vi "Initialize Sessions - NSess.vi"(6 "initialize and close session behavior":T1, 7 "option string":string, 8 "error in":errorcluster, 9 "reset":bool, 11 "session reservation in":refnum<class "Session Reservation.lvclass">) -> (0 "error out":errorcluster, 1 "channel lists":string[](array[string]), 2 "sessions":refnum<k15>[](array[refnum]), 3 "session reservation out":refnum<class "Session Reservation.lvclass">)   [LabVIEW 2020, in "MeasurementLink niDigital.lvlib"]
doc: "Create the NI-Digital driver sessions from the <b>session reservation in</b>."
uses:
  MeasurementLink niDigital.lvlib
  b3cb301c-7684-4518-818f-a956a366db36.vi
  Session Factory/Session Factory.lvclass
  Measurements/Measurement Plugin Session Management V1/Session Reservation/Session Reservation.lvclass
  Measurements/Measurement Plugin Session Management V1/Session Reservation/Initialize and Close Session Behavior.ctl
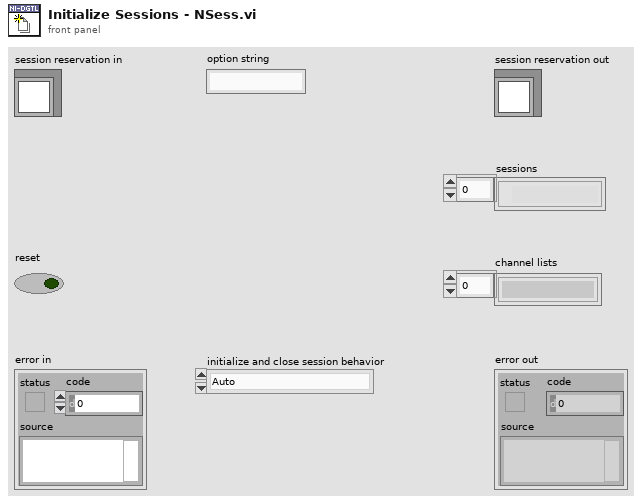
[diagram p1: front panel]
types:
  T1 = typedef "Measurement Plugin Session Management V1.lvlib/Session Reservation.lvclass/Initialize and Close Session Behavior.ctl" = enum16{"Auto", "Initialize and Close", "Attach and Detach", "Initialize and Detach", "Attach and Close"}
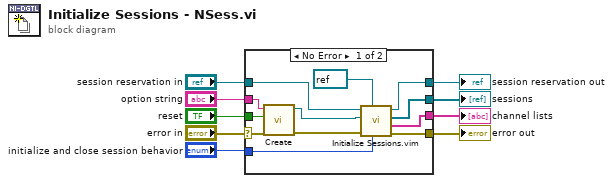
[diagram p0: block diagram]
diagram:
  n1 = case shown="No Error" "error in" {
    selector: "error in" -> [w15 w23]
    tunnel: [w19 w23] -> w8
    tunnel: [w20 w22] -> w6
    tunnel: "session reservation in" -> [w21 w22]
    tunnel: "option string" -> [w13 _]
    tunnel: "reset" -> [w14 _]
    tunnel: [w18 _] -> w3
    tunnel: [w17 _] -> w2
    tunnel: "initialize and close session behavior" -> [w10 _]
    frame No Error {
      n2 = call "Create.vi"("error in"=w15, "reset"=w14, "option string"=w13) -> ("error out"=w12:errorcluster, "session factory out"=w11:refnum<class "Session Factory.lvclass">)  [unwired: 7 in]
      n3 = call "Initialize Sessions.vim"("initialize and close session behavior"=w10, "session type"=refnum<k15> refnum ("instrument handle out"), "error in"=w12, "session factory"=w11, "session reservation in"=w21) -> ("error out"=w19:errorcluster, "channel lists"=w17:string[], "sessions"=w18:refnum<k15>[], "session reservation out"=w20:refnum<class "Session Reservation.lvclass">)  [unwired: 3 in]
    }
    frame Error {
    }
  }
  "error out" <- w8
  "session reservation out" <- w6
  "sessions" <- w3
  "channel lists" <- w2
